vi "RO PC.vi"() -> ()   [LabVIEW 2013]
doc: "Use this template to build a producer/consumer design pattern with events to produce queue items. Use this design pattern instead of the User Interface Event Handler pattern for user interfaces when you want to execute code asynchronously in response to an event without slowing the user interface responsiveness."
uses:
  RO PC.ctl
panel:
  out "Enum":T1
  out "Water":string
  in  "on/off":bool
  in  "Dispense":bool
  out "Indicator":cluster{"Red":bool, "Yellow":bool, "Green":bool}
  # "Red- Receive Water\nYellow-Process Water\nGreen- Ready to dispense\nwater"
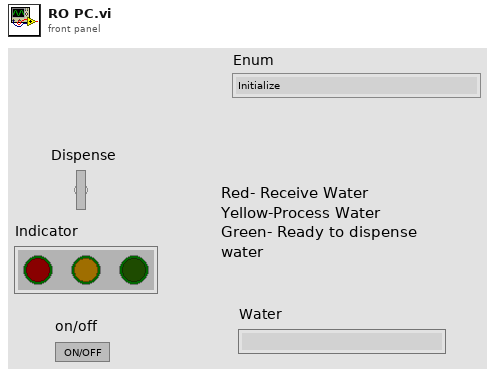
[diagram p1: front panel]
types:
  T1 = typedef "RO PC.ctl" = enum16{"Initialize", "Start", "Receive Water", "Process Water", "Signal water ready", "Dispense Water", "Stop"}
  T2 = enum8{"Enabled", "Disabled", "Disabled and Grayed Out"}
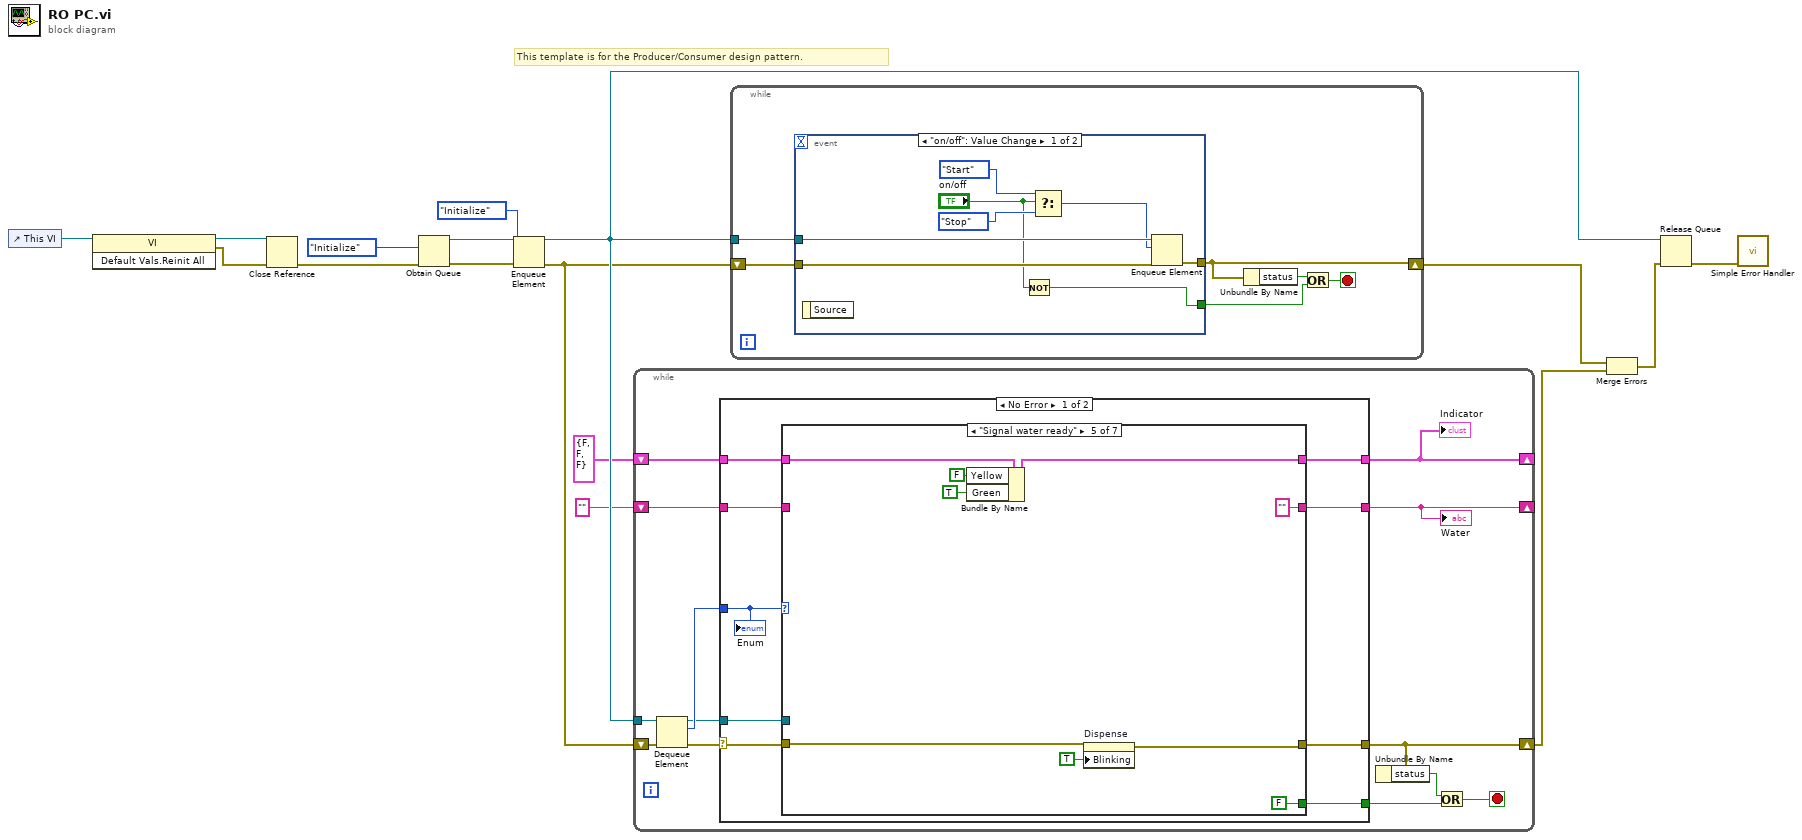
[diagram p0: block diagram]
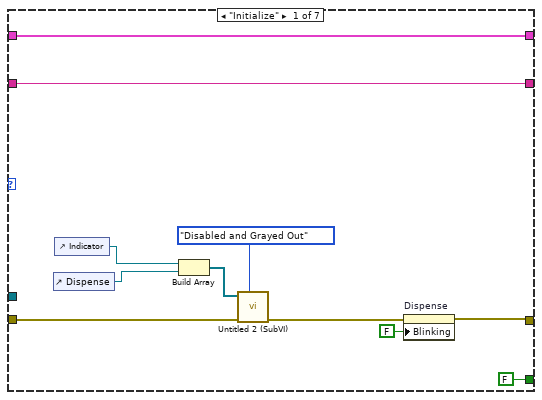
[diagram p2: hidden frame]
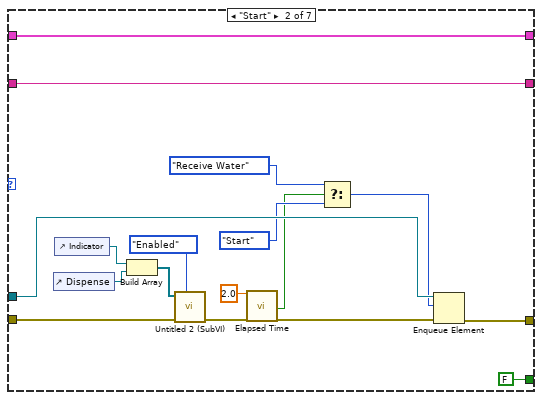
[diagram p3: hidden frame]
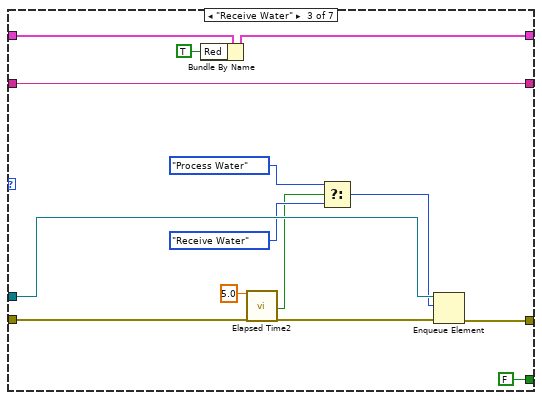
[diagram p4: hidden frame]
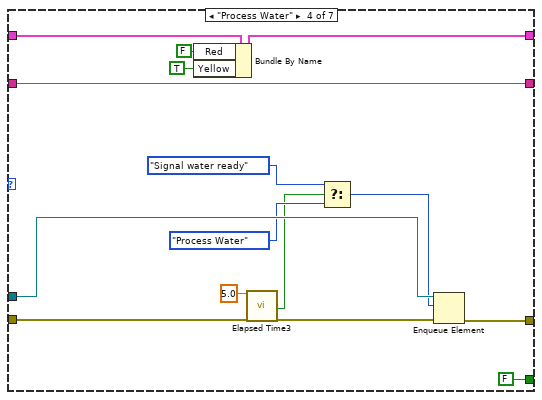
[diagram p5: hidden frame]
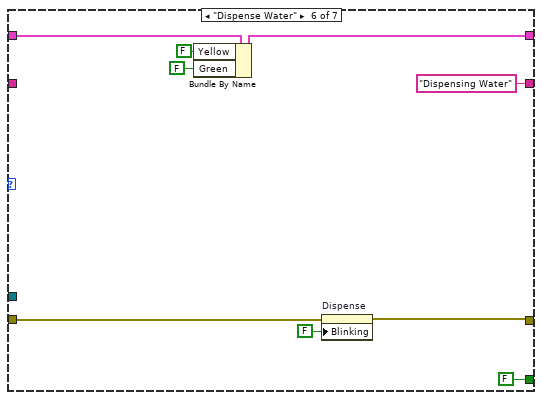
[diagram p6: hidden frame]
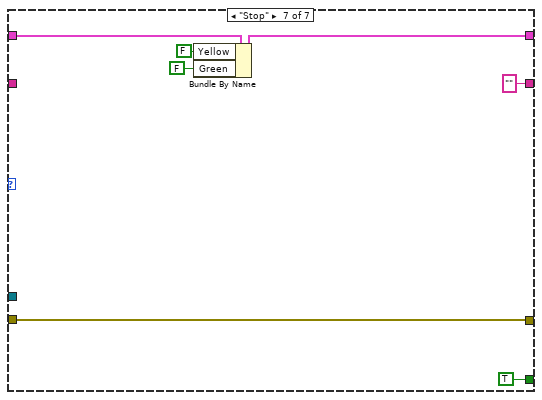
[diagram p7: hidden frame]
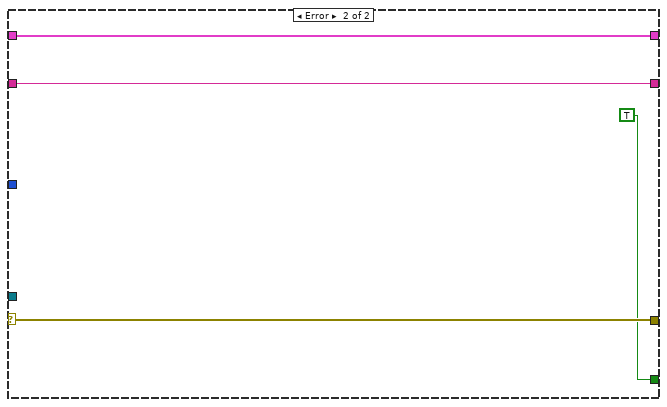
[diagram p8: hidden frame]
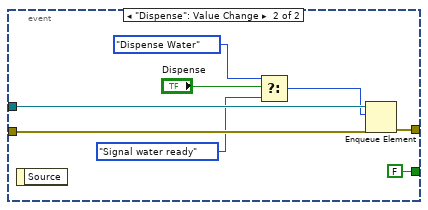
[diagram p9: hidden frame]
diagram:
  # "This template is for the Producer/Consumer design pattern."
  n1 = control-ref of="This VI"() -> (w16:refnum<vi>)
  n2 = invoke class="VI" method="Default Vals.Reinit All"(reference=w16) -> (reference out=w15:refnum<vi>, error out=w14:errorcluster)  [unwired: 2 in, 1 out]
  n3 = Close Reference(reference=w15, error in (no error)=w14) -> (error out=w5:errorcluster)
  n4 = Obtain Queue(element data type=RO_PC."Initialize", error in (no error)=w5) -> (queue out=w13:refnum<queue>, error out=w12:errorcluster)  [unwired: 3 in, 1 out]
  n5 = Enqueue Element(queue=w13, element=RO_PC."Initialize", error in (no error)=w12) -> (queue out=w11:refnum<queue>, error out=w4:errorcluster)  [unwired: 1 in, 1 out]
  n6 = while {
    tunnel: w11 -> [w29]
    shift-right: [w22] -> w6
    shift-left: w4 -> [w21]
    shift-right: [w19] -> _
    shift-left: cluster{"Red":bool, "Yellow":bool, "Green":bool} {"Red"=FALSE, "Yellow"=FALSE, "Green"=FALSE} ("Indicator") -> [w20]
    shift-right: [w17] -> _
    shift-left: "" ("f") -> [w18]
    stop <- w23 stop-if-true
    n7 = Dequeue Element(queue=w29, error in (no error)=w21) -> (queue out=w26:refnum<queue>, element=w28:T1, error out=w27:errorcluster)  [unwired: 1 in, 1 out]
    n8 = case shown="No Error" w27 {
      selector: w27 -> [w37 w124]
      tunnel: w28 -> [w38 _]
      tunnel: [w36 w124] -> w22
      tunnel: w26 -> [w35 _]
      tunnel: [w34 TRUE] -> w24
      tunnel: w20 -> [w33 w122]
      tunnel: [w32 w122] -> w19
      tunnel: [w31 w121] -> w17
      tunnel: w18 -> [w30 w121]
      frame No Error {
        n9 = case shown="\"Signal water ready\"" w38 {
          tunnel: w37 -> [w45 w62 w69 w84 w98 w107 w115]
          tunnel: [w40 w64 w80 w95 w97 w106 w115] -> w36
          tunnel: w35 -> [_ w61 w78 w93 _ _ _]
          tunnel: [FALSE FALSE FALSE FALSE FALSE FALSE TRUE] -> w34
          tunnel: w33 -> [w44 w60 w77 w92 w103 w112 w119]
          tunnel: [w44 w60 w68 w83 w102 w111 w118] -> w32
          tunnel: [w43 w59 w76 w91 "" ("f") "Dispensing Water" ("f") "" ("f")] -> w31
          tunnel: w30 -> [w43 w59 w76 w91 _ _ _]
          frame "Initialize" {
            n10 = control-ref of="Dispense"() -> (w48:refnum<vi>)
            n11 = control-ref of="Indicator"() -> (w49:refnum<vi>)
            n12 = Build Array(w49, w48) -> (w47:refnum<vi>[])
            n13 = call "Untitled 2 (SubVI).vi"("Disabled"=T2."Disabled and Grayed Out", "error in (no error)"=w45, "Array"=w47) -> ("error out"=w41:errorcluster)  [unwired: 8 in]
            n14 = property on="Dispense" class="Bool (strict)"(error in=w41, "Blinking"=FALSE) -> (error out=w40:errorcluster)  [unwired: 1 in, 1 out]
          }
          frame "Start" {
            n15 = control-ref of="Dispense"() -> (w65:refnum<vi>)
            n16 = control-ref of="Indicator"() -> (w66:refnum<vi>)
            n17 = Build Array(w66, w65) -> (w58:refnum<vi>[])
            n18 = call "Untitled 2 (SubVI).vi"("Disabled"=T2."Enabled", "error in (no error)"=w62, "Array"=w58) -> ("error out"=w57:errorcluster)  [unwired: 8 in]
            n19 = call "Elapsed Time"("Time Target (s)"=2.0, "error in (no error)"=w57) -> ("Time has Elapsed"=w52:bool, "error out"=w56:errorcluster)  [unwired: 10 in, 6 out]
            n20 = Select(t=RO_PC."Receive Water" ("element"), s=w52, f=RO_PC."Start" ("element")) -> (s? t:f=w51:T1)
            n21 = Enqueue Element(queue=w61, element=w51, error in (no error)=w56) -> (error out=w64:errorcluster)  [unwired: 1 in, 2 out]
          }
          frame "Receive Water" {
            n22 = Bundle By Name(cluster=w77, "Red"=TRUE) -> (w68:cluster{"Red":bool, "Yellow":bool, "Green":bool})
            n23 = call "Elapsed Time2"("Time Target (s)"=5.0, "error in (no error)"=w69) -> ("Time has Elapsed"=w71:bool, "error out"=w75:errorcluster)  [unwired: 10 in, 6 out]
            n24 = Select(t=RO_PC."Process Water" ("element"), s=w71, f=RO_PC."Receive Water" ("element")) -> (s? t:f=w70:T1)
            n25 = Enqueue Element(queue=w78, element=w70, error in (no error)=w75) -> (error out=w80:errorcluster)  [unwired: 1 in, 2 out]
          }
          frame "Process Water" {
            n26 = Bundle By Name(cluster=w92, "Red"=FALSE, "Yellow"=TRUE) -> (w83:cluster{"Red":bool, "Yellow":bool, "Green":bool})
            n27 = call "Elapsed Time3"("Time Target (s)"=5.0, "error in (no error)"=w84) -> ("Time has Elapsed"=w86:bool, "error out"=w90:errorcluster)  [unwired: 10 in, 6 out]
            n28 = Select(t=RO_PC."Signal water ready" ("element"), s=w86, f=RO_PC."Process Water" ("element")) -> (s? t:f=w85:T1)
            n29 = Enqueue Element(queue=w93, element=w85, error in (no error)=w90) -> (error out=w95:errorcluster)  [unwired: 1 in, 2 out]
          }
          frame "Signal water ready" {
            n30 = Bundle By Name(cluster=w103, "Yellow"=FALSE ("Red"), "Green"=TRUE ("Yellow")) -> (w102:cluster{"Red":bool, "Yellow":bool, "Green":bool})
            n31 = property on="Dispense" class="Bool (strict)"(error in=w98, "Blinking"=TRUE) -> (error out=w97:errorcluster)  [unwired: 1 in, 1 out]
          }
          frame "Dispense Water" {
            n32 = Bundle By Name(cluster=w112, "Yellow"=FALSE ("Red"), "Green"=FALSE ("Yellow")) -> (w111:cluster{"Red":bool, "Yellow":bool, "Green":bool})
            n33 = property on="Dispense" class="Bool (strict)"(error in=w107, "Blinking"=FALSE) -> (error out=w106:errorcluster)  [unwired: 1 in, 1 out]
          }
          frame "Stop" {
            n34 = Bundle By Name(cluster=w119, "Yellow"=FALSE ("Red"), "Green"=FALSE ("Yellow")) -> (w118:cluster{"Red":bool, "Yellow":bool, "Green":bool})
          }
        }
        "Enum" <- w38
      }
      frame Error {
      }
    }
    "Indicator" <- w19
    "Water" <- w17
    n35 = Unbundle By Name(w22) -> ("status"=w25:bool)
    n36 = Or(x=w25, y=w24) -> (x .or. y?=w23:bool)
  }
  n37 = while {
    shift-right: [w127] -> w8
    shift-left: w4 -> [w129]
    tunnel: w11 -> [w130]
    stop <- w128 stop-if-true
    n38 = event shown="[0] \"on/off\": Value Change" {
      selector: _ -> [_ _]
      dyn-events: _ -> [_ _]
      timeout: _ -> [_ _]
      tunnel: w130 -> [w138 w146]
      tunnel: w129 -> [w137 w145]
      tunnel: [w136 w144] -> w127
      tunnel: [w131 FALSE] -> w125
      event "on/off": Value Change {
        n39 = event-data() -> ()  [unwired: 1 in, 1 out]
        n40 = Not(x="on/off") -> (.not. x?=w131:bool)
        n41 = Select(t=RO_PC."Start" ("element"), s="on/off", f=RO_PC."Stop" ("element")) -> (s? t:f=w133:T1)
        n42 = Enqueue Element(queue=w138, element=w133, error in (no error)=w137) -> (error out=w136:errorcluster)  [unwired: 1 in, 2 out]
      }
      event "Dispense": Value Change {
        n43 = event-data() -> ()  [unwired: 1 in, 1 out]
        n44 = Select(t=RO_PC."Dispense Water" ("element"), s="Dispense", f=RO_PC."Signal water ready" ("element")) -> (s? t:f=w141:T1)
        n45 = Enqueue Element(queue=w146, element=w141, error in (no error)=w145) -> (error out=w144:errorcluster)  [unwired: 1 in, 2 out]
      }
    }
    n46 = Unbundle By Name(w127) -> ("status"=w126:bool)
    n47 = Or(x=w126, y=w125) -> (x .or. y?=w128:bool)
  }
  n48 = Merge Errors(w8, w6) -> (w7:errorcluster)
  n49 = Release Queue(queue=w11, error in (no error)=w7) -> (error out=w3:errorcluster)  [unwired: 1 in, 2 out]
  n50 = call <vilib>:"Simple Error Handler.vi"("error in (no error)"=w3) -> ()  [unwired: 4 in, 5 out]
